vi "SDT_WriteFile.vi"(4 "adc_re[dig]":i16=256, 5 "ActiveModule":string[](array[string]), 7 "Data":T12, 8 "ErrorIn":errorcluster, 9 "SPCdata":T13={"base_adr"=52672, "init"=0, "cfd_limit_low"=-0.0, "cfd_limit_high"=5.019608, "cfd_zc_level"=-5.2913384, "cfd_holdoff"=5.0, "sync_zc_level"=-5.2913384, "sync_holdoff"=4.0, "sync_threshold"=-70.588234, "tac_range"=50.033573, "sync_freq_div"=1, "tac_gain"=1, "tac_offset"=5.098039, "tac_limit_low"=0.0, "tac_limit_high"=100.0, "adc_resolution"=12, "ext_latch_delay"=0, "collect_time"=1.0, "display_time"=1.0, "repeat_time"=10.0, "stop_on_time"=1, "stop_on_ovfl"=1, "dither_range"=128, "count_incr"=1, "mem_bank"=0, "dead_time_comp"=0, "scan_control"=0, "routing_mode"=0, "tac_enable_hold"=0.0, "pci_card_no"=-1, "mode"=5, "scan_size_x"=1, "scan_size_y"=1, "scan_rout_x"=1, "scan_rout_y"=1, "scan_flyback"=65537, "scan_borders"=0, "scan_polarity"=0, "pixel_clock"=1, "line_compression"=1, "trigger"=0, "pixel_time"=1e-07, "ext_pixclk_div"=1, "rate_count_time"=1.0, "macro_time_clk"=0, "add_select"=0, "test_eep"=1, "adc_zoom"=0, "img_size_x"=1, "img_size_y"=1, "img_rout_x"=1, "img_rout_y"=1, "xy_gain"=1, "master_clock"=0, "adc_sample_delay"=0, "detector_type"=1, "chan_enable"=4191231, "chan_slope"=0, "chan_spec_no"=34835, "tdc_control"=0, "tdc_offset1"=0.0, "tdc_offset2"=0.0, "tdc_offset3"=0.0, "tdc_offset4"=0.0, "future_reserve1"=0, "future_reserve2"=0, "future_reserve3"=0, "future_reserve4"=0, "future_reserve5"=0, "future_reserve6"=0, "future_reserve7"=0} {"scan_flyback" format="%x"}, 10 "ImageSize":i32=256, 11 "SDT-FilePath":path=path "\\\\lab13\\C/Users/jannis/Desktop/ZeissFifo.sdt") -> (0 "ErrorOut":errorcluster)   [LabVIEW 2019]
doc: "This VI writes a SDT-file to disc. The SetUp and the MeasureInfo blocks are created and appended with the data blocks. \nThis VI is limited to writing a DecayMatrix from a FIFO-Image recording and optional an IntensityImage to file. For single mode recordings use the spcmdll VI \\Public\\Configure\\Memory Transfer\\SPC_save_data_to_sdtfile.vi.\nFor a description of the format for the Data input cluster to this VI see the usage in \\Example\\ImagingEventStream-SimpleFifoImage.vi. Leave either of the cluster input arrays empty to not save them to disc.\nFor a description of the *.sdt file format see: SPC_data_file_structure.h\n\ninfo@becker-hickl.com"
uses:
  SPC_Controls/FileType.ctl
  SPC_Controls/bhfile_header.ctl
  SPC_Controls/SPCdata.ctl
  SPC_Controls/MeasureInfo_PartB.ctl
  SPC_Controls/MeasStopInfo.ctl
  SPC_Controls/MeasFCSInfo.ctl
  SPC_Controls/MeasureInfo_PartE.ctl
  SPC_Controls/MeasHISTInfo.ctl
  SPC_Controls/HISTInfoExt.ctl
  SPC_Controls/MeasureInfo_PartI.ctl
  SPC_Controls/MeasureInfo_PartK.ctl
  SPC_Controls/MeasureInfo_PartM.ctl
  SPC_Controls/MeasureInfo.ctl
  SPC_Controls/BHFileBlockHeader.ctl
panel:
  out "Info Block":string
  out "BHFileBlockHeaders":T1[](array[typedef])
  out "MeasureInfos":T2[](array[typedef]) {"MeasStopInfo"."flags" format="x%x"}
  out "BlockLengths":i32[](array[numeric])
  out "bhfile_header":T14 {"chksum" format="x%x"; "header_valid" format="x%x"}
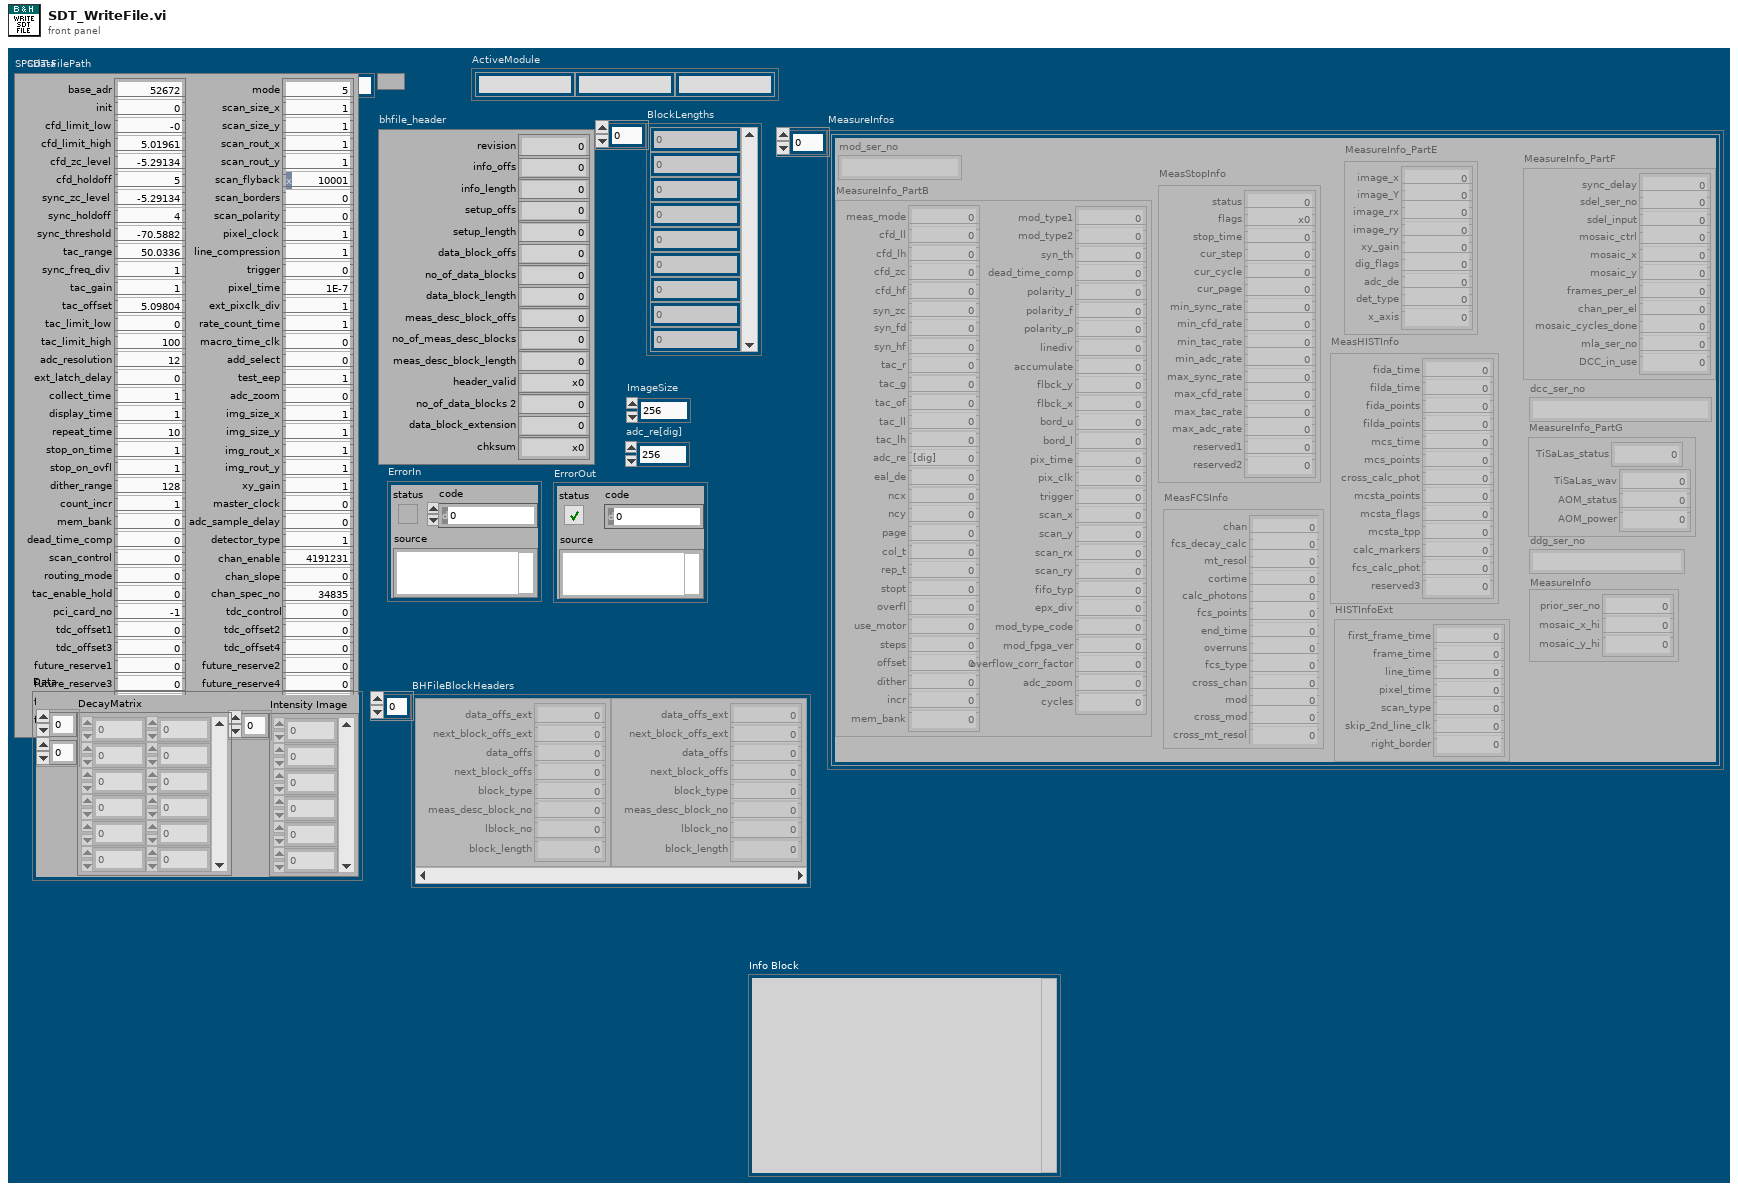
[diagram p1: front panel]
types:
  T1 = typedef "BHFileBlockHeader.ctl" = cluster{"data_offs_ext":u8, "next_block_offs_ext":u8, "data_offs":u32, "next_block_offs":u32, "block_type":u16, "meas_desc_block_no":i16, "lblock_no":u32, "block_length":u32}
  T2 = typedef "MeasureInfo.ctl" = cluster{"mod_ser_no":string, "MeasureInfo_PartB":T3, "MeasStopInfo":T4, "MeasFCSInfo":T5, "MeasureInfo_PartE":T6, "MeasHISTInfo":T7, "HISTInfoExt":T8, "MeasureInfo_PartF":T9, "dcc_ser_no":string, "MeasureInfo_PartG":T10, "ddg_ser_no":string, "MeasureInfo":T11}
  T3 = typedef "MeasureInfo_PartB.ctl" = cluster{"meas_mode":i16, "cfd_ll":sgl, "cfd_lh":sgl, "cfd_zc":sgl, "cfd_hf":sgl, "syn_zc":sgl, "syn_fd":i16, "syn_hf":sgl, "tac_r":sgl, "tac_g":i16, "tac_of":sgl, "tac_ll":sgl, "tac_lh":sgl, "adc_re":i16, "eal_de":i16, "ncx":i16, "ncy":i16, "page":u16, "col_t":sgl, "rep_t":sgl, "stopt":i16, "overfl":i8, "use_motor":i16, "steps":u16, "offset":sgl, "dither":i16, "incr":i16, "mem_bank":i16, "mod_type1":u64, "mod_type2":u64, "syn_th":sgl, "dead_time_comp":i16, "polarity_l":i16, "polarity_f":i16, "polarity_p":i16, "linediv":i16, "accumulate":i16, "flbck_y":i32, "flbck_x":i32, "bord_u":i32, "bord_l":i32, "pix_time":sgl, "pix_clk":i16, "trigger":i16, "scan_x":i32, "scan_y":i32, "scan_rx":i32, "scan_ry":i32, "fifo_typ":i16, "epx_div":i32, "mod_type_code":u16, "mod_fpga_ver":u16, "overflow_corr_factor":sgl, "adc_zoom":i32, "cycles":i32}
  T4 = typedef "MeasStopInfo.ctl" = cluster{"status":u16, "flags":u16, "stop_time":sgl, "cur_step":i32, "cur_cycle":i32, "cur_page":i32, "min_sync_rate":sgl, "min_cfd_rate":sgl, "min_tac_rate":sgl, "min_adc_rate":sgl, "max_sync_rate":sgl, "max_cfd_rate":sgl, "max_tac_rate":sgl, "max_adc_rate":sgl, "reserved1":i32, "reserved2":sgl}
  T5 = typedef "MeasFCSInfo.ctl" = cluster{"chan":u16, "fcs_decay_calc":u16, "mt_resol":u32, "cortime":sgl, "calc_photons":u32, "fcs_points":i32, "end_time":sgl, "overruns":u16, "fcs_type":u16, "cross_chan":u16, "mod":u16, "cross_mod":u16, "cross_mt_resol":u32}
  T6 = typedef "MeasureInfo_PartE.ctl" = cluster{"image_x":i32, "image_Y":i32, "image_rx":i32, "image_ry":i32, "xy_gain":i16, "dig_flags":i16, "adc_de":i16, "det_type":i16, "x_axis":i16}
  T7 = typedef "MeasHISTInfo.ctl" = cluster{"fida_time":sgl, "filda_time":sgl, "fida_points":i32, "filda_points":i32, "mcs_time":sgl, "mcs_points":i32, "cross_calc_phot":u32, "mcsta_points":u16, "mcsta_flags":u16, "mcsta_tpp":u32, "calc_markers":u32, "fcs_calc_phot":u32, "reserved3":u32}
  T8 = typedef "HISTInfoExt.ctl" = cluster{"first_frame_time":sgl, "frame_time":sgl, "line_time":sgl, "pixel_time":sgl, "scan_type":i16, "skip_2nd_line_clk":i16, "right_border":u32}
  T9 = typedef "MeasureInfo_PartI.ctl" = cluster{"sync_delay":sgl, "sdel_ser_no":u16, "sdel_input":i8, "mosaic_ctrl":i8, "mosaic_x":u8, "mosaic_y":u8, "frames_per_el":i16, "chan_per_el":i16, "mosaic_cycles_done":i32, "mla_ser_no":u16, "DCC_in_use":u8}
  T10 = typedef "MeasureInfo_PartK.ctl" = cluster{"TiSaLas_status":u16, "TiSaLas_wav":u16, "AOM_status":u8, "AOM_power":u8}
  T11 = typedef "MeasureInfo_PartM.ctl" = cluster{"prior_ser_no":i32, "mosaic_x_hi":u8, "mosaic_y_hi":u8}
  T12 = cluster{"DecayMatrix":u16[][], "Intensity Image":u32[]}
  T13 = typedef "SPCdata.ctl" = cluster{"base_adr":u16, "init":i16, "cfd_limit_low":sgl, "cfd_limit_high":sgl, "cfd_zc_level":sgl, "cfd_holdoff":sgl, "sync_zc_level":sgl, "sync_holdoff":sgl, "sync_threshold":sgl, "tac_range":sgl, "sync_freq_div":i16, "tac_gain":i16, "tac_offset":sgl, "tac_limit_low":sgl, "tac_limit_high":sgl, "adc_resolution":i16, "ext_latch_delay":i16, "collect_time":sgl, "display_time":sgl, "repeat_time":sgl, "stop_on_time":i16, "stop_on_ovfl":i16, "dither_range":i16, "count_incr":i16, "mem_bank":i16, "dead_time_comp":i16, "scan_control":u16, "routing_mode":u16, "tac_enable_hold":sgl, "pci_card_no":i16, "mode":u16, "scan_size_x":u32, "scan_size_y":u32, "scan_rout_x":u32, "scan_rout_y":u32, "scan_flyback":u32, "scan_borders":u32, "scan_polarity":u16, "pixel_clock":u16, "line_compression":u16, "trigger":u16, "pixel_time":sgl, "ext_pixclk_div":u32, "rate_count_time":sgl, "macro_time_clk":i16, "add_select":i16, "test_eep":i16, "adc_zoom":i16, "img_size_x":u32, "img_size_y":u32, "img_rout_x":u32, "img_rout_y":u32, "xy_gain":i16, "master_clock":i16, "adc_sample_delay":i16, "detector_type":i16, "chan_enable":u32, "chan_slope":u32, "chan_spec_no":u32, "tdc_control":u32, "tdc_offset1":sgl, "tdc_offset2":sgl, "tdc_offset3":sgl, "tdc_offset4":sgl, "future_reserve1":u64, "future_reserve2":u64, "future_reserve3":u64, "future_reserve4":u64, "future_reserve5":u64, "future_reserve6":u64, "future_reserve7":u64}
  T14 = typedef "bhfile_header.ctl" = cluster{"revision":i16, "info_offs":i32, "info_length":i16, "setup_offs":i32, "setup_length":u16, "data_block_offs":i32, "no_of_data_blocks":i16, "data_block_length":u32, "meas_desc_block_offs":i32, "no_of_meas_desc_blocks":i16, "meas_desc_block_length":i16, "header_valid":u16, "no_of_data_blocks 2":u32, "data_block_extension":u16, "chksum":u16}
  T15 = typedef "FileType.ctl" = u16
  T16 = enum16{"open", "replace", "create", "open or create", "replace or create", "replace or create with confirmation"}
  T17 = enum16{"big-endian, network order", "native, host order", "little-endian"}
  T18 = typedef "BHModuleType.ctl" = i16
  T19 = typedef "ModuleType.ctl" = i16
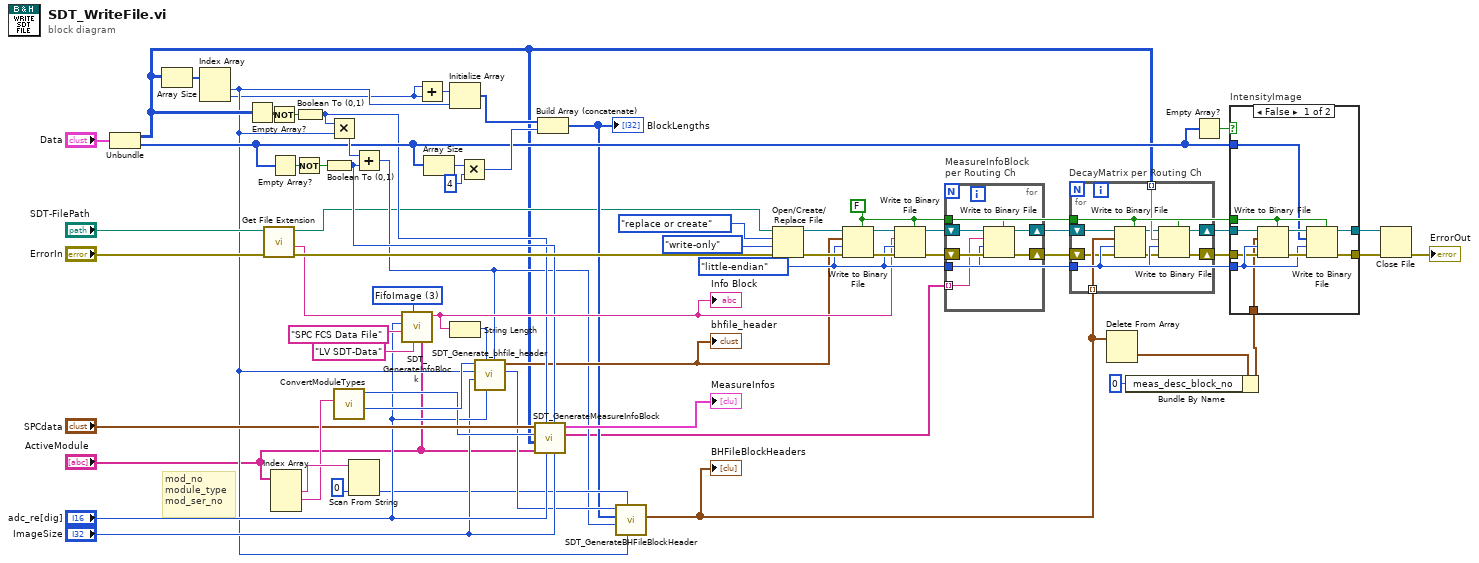
[diagram p0: block diagram]
diagram:
  w2 = T15 3 items=["non-Fifo"=1, "Fifo"=2, "FifoImage"=3] ("FileType")
  w55 = FALSE ("prepend array or string size? (T)")
  w54 = T17."little-endian" ("byte order (0:big-endian, network order)")
  # "mod_no\nmodule_type\nmod_ser_no"
  n1 = Unbundle("Data") -> ("DecayMatrix"=w5:u16[][], "Intensity Image"=w28:u32[])
  n2 = Array Size(array=w5) -> (size(s)=w37:i32[])
  n3 = Index Array(array=w37) -> (element #1=w4:i32, element #2=w3:i32)  [unwired: 2 in]
  n4 = Empty Array?(array=w5) -> (empty?=w47:bool)
  n5 = call <vilib>:"Get File Extension.vi"("error in (no error)"="ErrorIn", "file"="SDT-FilePath") -> ("error out"=w61:errorcluster, "filename without extension"=w27:string, "dup file"=w7:path)  [unwired: 5 in, 2 out]
  n6 = Not(x=w47) -> (.not. x?=w45:bool)
  n7 = Empty Array?(array=w28) -> (empty?=w46:bool)
  n8 = Index Array(array="ActiveModule") -> (element #1=w43:string, element #2=w39:string)  [unwired: 3 in, 1 out]
  n9 = Not(x=w46) -> (.not. x?=w44:bool)
  n10 = Boolean To (0,1)(Boolean=w45) -> (0, 1=w15:i16)
  n11 = Boolean To (0,1)(Boolean=w44) -> (0, 1=w20:i16)
  n12 = Multiply(x=w15, y=w4) -> (x*y=w34:i32)
  n13 = call "ConvertModuleTypes.vi"("ModuleTypeStringIn"=w39) -> ("BHModuleType"=w22:T18, "Module TypeOut"=w19:T19)  [unwired: 8 in, 1 out]
  n14 = Scan From String(input string=w43, default 1=u32 0 ("meas_desc_block_no")) -> (output 1=w11:u32)  [unwired: 3 in, 3 out]
  n15 = Add(x=w34, y=w20) -> (x+y=w9:i32)
  n16 = call "SDT_GenerateInfoBlock.vi"("ActiveModule"="ActiveModule", "Contents"="LV SDT-Data", "FileType"=w2, "FileID"="SPC FCS Data File", "adc_re[dig]"="adc_re[dig]", "FilenameNoExtension"=w27) -> ("Info Block"=w24:string)  [unwired: 5 in]
  "Info Block" <- w24
  n17 = Add(x=w3, y=w3) -> (x+y=w36:i32)
  n18 = Array Size(array=w28) -> (size(s)=w49:i32)
  n19 = Initialize Array(w36, w4) -> (w35:i32[])
  n20 = String Length(string=w24) -> (length=w23:i32)
  n21 = Multiply(x=w49, y=4) -> (x*y=w41:i32)
  n22 = call "SDT_Generate_bhfile_header.vi"("no_of_data_blocks"=w9, "adc_re[dig]"="adc_re[dig]", "info_length"=w23, "ImageSize"="ImageSize", "NoOfRoutingChannel"=w4, "BHModuleType"=w22) -> ("data_block_offs"=w12:i32, "bhfile_header"=w14:T14)  [unwired: 4 in]
  "bhfile_header" <- w14
  n23 = call "SDT_GenerateMeasureInfoBlock.vi"("ImageSize"="ImageSize", "HasIntensityImage"=w20, "adc_re[dig]"="adc_re[dig]", "HasFifoImage"=w15, "ActiveModule"="ActiveModule", "DecayMatrix"=w5, "Module Type"=w19, "SPCdata"="SPCdata") -> ("MeasureInfoStrings"=w6:string[], "MeasureInfos"=→"MeasureInfos":T2[])  [unwired: 2 in]
  n24 = Build Array (concatenate)(w35, w41) -> (w10:i32[])
  "BlockLengths" <- w10
  n25 = call "SDT_GenerateBHFileBlockHeader.vi"("NoOfRoutingChannels"=w4, "ModuleNo"=w11, "NoOfDataBlocks"=w9, "BlockLengths"=w10, "data_block_offs"=w12) -> ("BHFileBlockHeaders"=w13:T1[])  [unwired: 5 in, 1 out]
  "BHFileBlockHeaders" <- w13
  n26 = Open/Create/Replace File(file path (use dialog)=w7, error in=w61, operation (0:open)=T16."replace or create", access (0:read/write)=enum16{"read/write", "read-only", "write-only"}."write-only") -> (refnum out=w64:refnum<file>, error out=w60:errorcluster)  [unwired: 2 in, 1 out]
  n27 = Write to Binary File(file (use dialog)=w64, data=w14, error in=w60, 5:w55, 9:w54) -> (refnum out=w63:refnum<file>, error out=w59:errorcluster)  [unwired: 1 in, 1 out]
  n28 = Write to Binary File(file (use dialog)=w63, data=w24, error in=w59, 5:w55, 9:w54) -> (refnum out=w62:refnum<file>, error out=w58:errorcluster)  [unwired: 1 in, 1 out]
  n29 = for "MeasureInfoBlock\nper Routing Ch" {
    tunnel: w55 -> [w71]
    tunnel: w54 -> [w70]
    shift-right: [w69] -> w33
    shift-left: w62 -> [w73]
    shift-right: [w68] -> w32
    shift-left: w58 -> [w72]
    tunnel: w6 -> [w67] mode=indexing
    n30 = Write to Binary File(file (use dialog)=w73, data=w67, error in=w72, 5:w71, 9:w70) -> (refnum out=w69:refnum<file>, error out=w68:errorcluster)  [unwired: 1 in, 1 out]
  }
  n31 = for "DecayMatrix per Routing Ch" {
    tunnel: w55 -> [w83]
    tunnel: w54 -> [w82]
    tunnel: w13 -> [w79] mode=indexing
    tunnel: w5 -> [w78] mode=indexing
    shift-right: [w80] -> w52
    shift-left: w33 -> [w77]
    shift-right: [w81] -> w53
    shift-left: w32 -> [w76]
    n32 = Write to Binary File(file (use dialog)=w77, data=w79, error in=w76, 5:w83, 9:w82) -> (refnum out=w75:refnum<file>, error out=w74:errorcluster)  [unwired: 1 in, 1 out]
    n33 = Write to Binary File(file (use dialog)=w75, data=w78, error in=w74, 5:w83, 9:w82) -> (refnum out=w80:refnum<file>, error out=w81:errorcluster)  [unwired: 1 in, 1 out]
  }
  n34 = Delete From Array(array=w13) -> (deleted portion=w38:T1)  [unwired: 2 in, 1 out]
  n35 = Bundle By Name(cluster=w38, "meas_desc_block_no"=i16 0) -> (w31:T1)
  n36 = Empty Array?(array=w28) -> (empty?=w29:bool)
  n37 = case "IntensityImage" shown="False" w29 {
    tunnel: w55 -> [w91 _]
    tunnel: w54 -> [w90 _]
    tunnel: w53 -> [w89 w94]
    tunnel: w52 -> [w88 w95]
    tunnel: [w87 w94] -> w51
    tunnel: [w86 w95] -> w50
    tunnel: w28 -> [w85 _]
    tunnel: w31 -> [w84 _]
    frame False {
      n38 = Write to Binary File(file (use dialog)=w88, data=w84, error in=w89, 5:w91, 9:w90) -> (refnum out=w92:refnum<file>, error out=w93:errorcluster)  [unwired: 1 in, 1 out]
      n39 = Write to Binary File(file (use dialog)=w92, data=w85, error in=w93, 5:w91, 9:w90) -> (refnum out=w86:refnum<file>, error out=w87:errorcluster)  [unwired: 1 in, 1 out]
    }
    frame True {
    }
  }
  n40 = Close File(refnum=w50, error in=w51) -> (error out=→"ErrorOut":errorcluster)  [unwired: 1 out]
